vi "LoadNodeUI.vi"(7 "user event out":T1, 8 "error in":errorcluster, 9 "sub panel ref in":refnum<vi>, 10 "main queue":T3, 11 "node":T2) -> (0 "error out":errorcluster)   [LabVIEW 2013, in "NISE_CEF_TreeControl.lvlib"]
doc: "This VI will insert the UI from a node into a subpanel."
uses:
  NISE_CEF_TreeControl.lvlib
  <vilib>/NI/AMC/Message Queue.ctl
  <vilib>/NI/AMC/Message.ctl
  <vilib>/NI/Tools/Keyed Array/KeyedArray.ctl
  Node/NodeRef.ctl
  Node/NISE_CEF_Node.lvclass
  Node/UserEventRef.ctl
  Controls/EventCluster.ctl
  <vilib>/NI/Tools/Keyed Array/Tools_KeyedArray.lvlib
  <vilib>/NI/AMC/AMC.lvlib
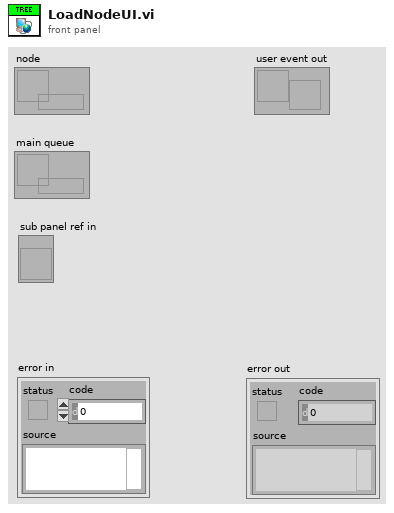
[diagram p1: front panel]
types:
  T1 = typedef "NISE_CEF_Node.lvclass/UserEventRef.ctl" = refnum<user-event>
  T2 = typedef "NISE_CEF_Node.lvclass/NodeRef.ctl" = refnum<data-value>
  T3 = typedef "AMC.lvlib/Message Queue.ctl" = refnum<queue>
  T4 = enum32{"Bad", "Idle", "Run top level", "Running"}
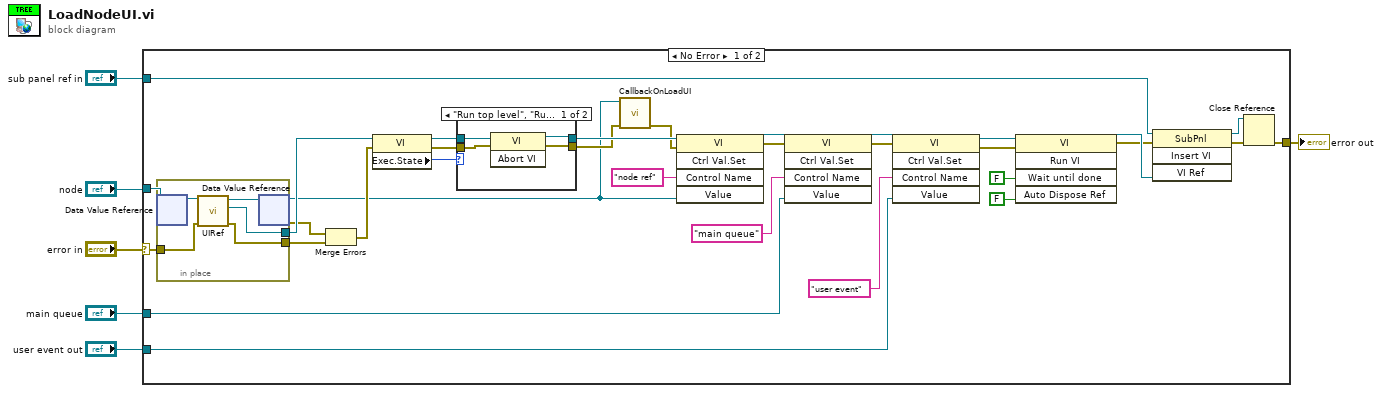
[diagram p0: block diagram]
diagram:
  n1 = case shown="No Error" "error in" {
    selector: "error in" -> [w22 w50]
    tunnel: [w28 w50] -> w5
    tunnel: "node" -> [w16 _]
    tunnel: "main queue" -> [w15 _]
    tunnel: "user event out" -> [w14 _]
    tunnel: "sub panel ref in" -> [w13 _]
    frame No Error {
      n2 = in-place {
        in-place-border: w22 -> [w46]
        in-place-border: [w47] -> w21
        in-place-border: [w45] -> w12
        n3 = in-place-dvr #1(w16) -> (w49:refnum<class "NISE_CEF_Node.lvclass">)  [unwired: 1 out]
        n4 = call-dynamic "UIRef.vi"("error in"=w46, "node in"=w49) -> ("error out"=w45:errorcluster, "VI refnum"=w47:refnum<vi>, "node out"=w48:refnum<class "NISE_CEF_Node.lvclass">)  [unwired: 7 in]
        n5 = in-place-dvr #1(w48) -> (w7:T2, w11:errorcluster)
      }
      n6 = Merge Errors(w11, w12) -> (w10:errorcluster)
      n7 = property class="VI"(reference=w21, error in=w10) -> (reference out=w18:refnum<vi>, error out=w17:errorcluster, "Exec.State"=w20:T4)
      n8 = case shown="\"Run top level\", \"Running\"" w20 {
        tunnel: [w39 w44] -> w19
        tunnel: w18 -> [w42 w44]
        tunnel: w17 -> [w41 w43]
        tunnel: [w40 w43] -> w9
        frame "Run top level", "Running" {
          n9 = invoke class="VI" method="Abort VI"(reference=w42, error in=w41) -> (reference out=w39:refnum<vi>, error out=w40:errorcluster)  [unwired: 1 in, 1 out]
        }
        frame "Idle", Default {
        }
      }
      n10 = call "CallbackOnLoadUI.vi"("error in"=w9, "node"=w7) -> ("error out"=w8:errorcluster)  [unwired: 9 in]
      n11 = invoke class="VI" method="Ctrl Val.Set"(reference=w19, error in=w8, "Control Name"="node ref", "Value"=w7) -> (reference out=w36:refnum<vi>, error out=w31:errorcluster)  [unwired: 1 in, 3 out]
      n12 = invoke class="VI" method="Ctrl Val.Set"(reference=w36, error in=w31, "Control Name"="main queue", "Value"=w15) -> (reference out=w26:refnum<vi>, error out=w27:errorcluster)  [unwired: 1 in, 3 out]
      n13 = invoke class="VI" method="Ctrl Val.Set"(reference=w26, error in=w27, "Control Name"="user event", "Value"=w14) -> (reference out=w25:refnum<vi>, error out=w24:errorcluster)  [unwired: 1 in, 3 out]
      n14 = invoke class="VI" method="Run VI"(reference=w25, error in=w24, "Wait until done"=FALSE ("Wait Until Done"), "Auto Dispose Ref"=FALSE ("Auto Dispose Reference")) -> (reference out=w35:refnum<vi>, error out=w34:errorcluster)  [unwired: 1 in, 3 out]
      n15 = invoke class="SubPnl" method="Insert VI"(reference=w13, error in=w34, "VI Ref"=w35) -> (reference out=w29:refnum<vi>, error out=w30:errorcluster)  [unwired: 1 in, 2 out]
      n16 = Close Reference(reference=w29, error in (no error)=w30) -> (error out=w28:errorcluster)
    }
    frame Error {
    }
  }
  "error out" <- w5
